vi "PJT_14.vi"() -> ()   [LabVIEW 2019]
panel:
  in  "정지":bool
  out "웨이브폼 차트":dbl(graph)
  in  "다이얼":dbl(knob) scale=0.0..100.0
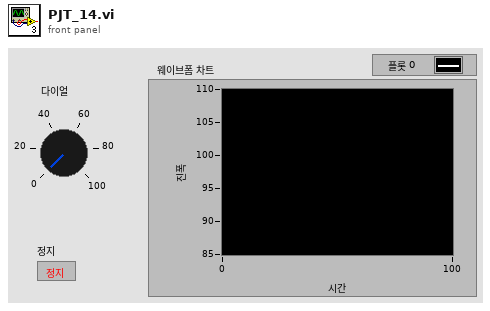
[diagram p1: front panel]
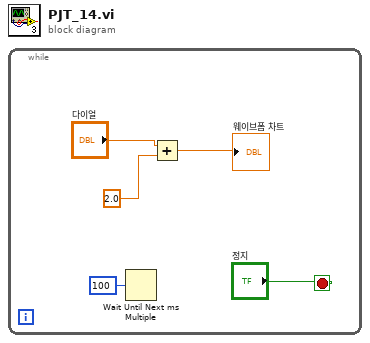
[diagram p0: block diagram]
diagram:
  n1 = while {
    stop <- "정지" stop-if-true
    n2 = Wait Until Next ms Multiple(millisecond multiple=u32 100 ("ms 배수")) -> ()  [unwired: 1 out]
    n3 = Add(x="다이얼", y=2.0) -> (x+y=→"웨이브폼 차트":dbl)
  }
